vi "Detect Connected Chassis.vi"(8 "error in":errorcluster, 11 "Refnum in":refnum<k21>) -> (0 "error out":errorcluster, 2 "Chassis Information":T1[](array[typedef]) {"Modules"."Module Code" format="%.0x"})   [LabVIEW 2015, in "SMI.lvlib" / "Controller.lvclass"]
uses:
  Controller.lvclass
  Chassis/Controls/ChassisInformation.ctl
  Module/Controls/ModuleInformation.ctl
  <vilib>/nisyscfg/Close (Resources).vi
  <vilib>/nisyscfg/Close (Filter).vi
  <vilib>/nisyscfg/Close (System).vi
  <vilib>/nisyscfg/nisyscfg.lvlib
  <resource>/objmgr/niflexriosae.rc
  <resource>/objmgr/nisysapi.rc
  Module/Module.lvclass
  Chassis/Chassis.lvclass
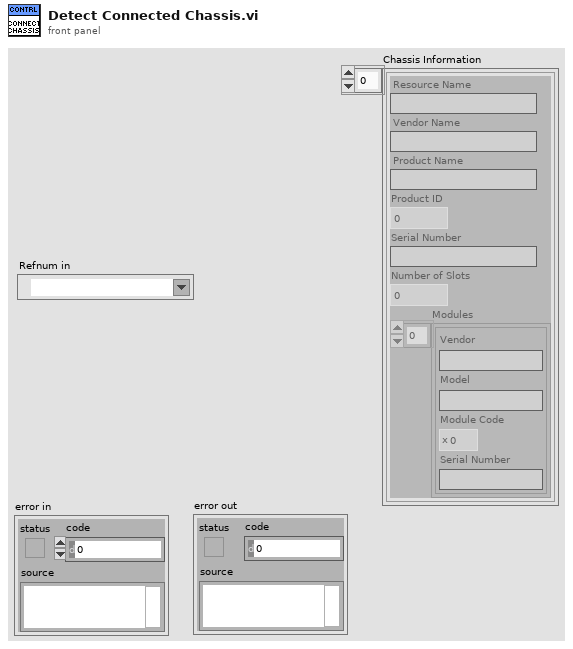
[diagram p1: front panel]
types:
  T1 = typedef "SMI.lvlib/Chassis.lvclass/ChassisInformation.ctl" = cluster{"Resource Name":string, "Vendor Name":string, "Product Name":string, "Product ID":u32, "Serial Number":string, "Number of Slots":i32, "Modules":T2[]}
  T2 = typedef "SMI.lvlib/Module.lvclass/ModuleInformation.ctl" = cluster{"Vendor":string, "Model":string, "Module Code":u32, "Serial Number":string}
  T3 = cluster{"VendorName":string, "ProdName":string, "SerialNum":string, "NumSlots":i32, "ProdID":u32, "Resource Name":string}
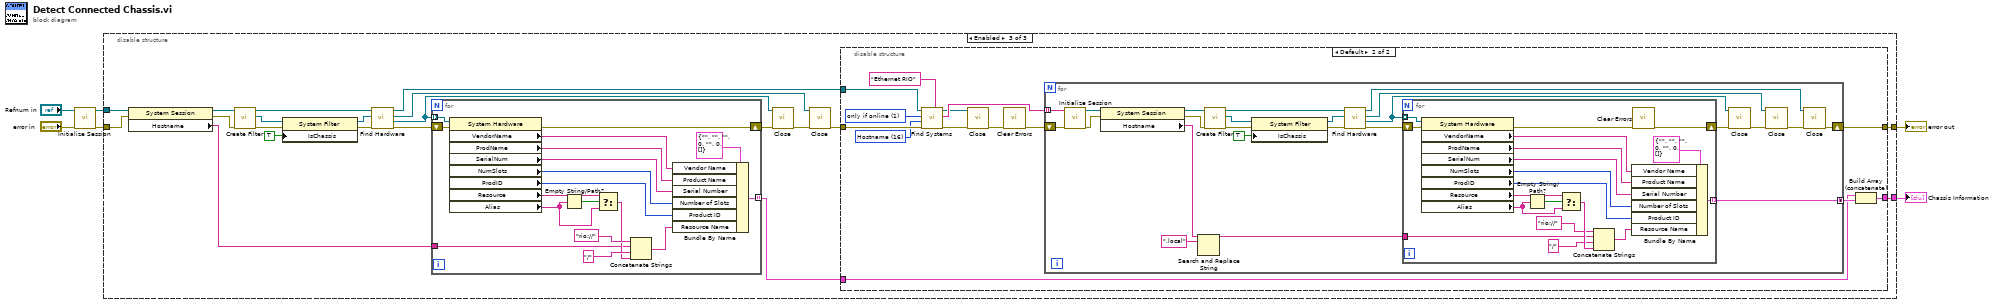
[diagram p0: block diagram]
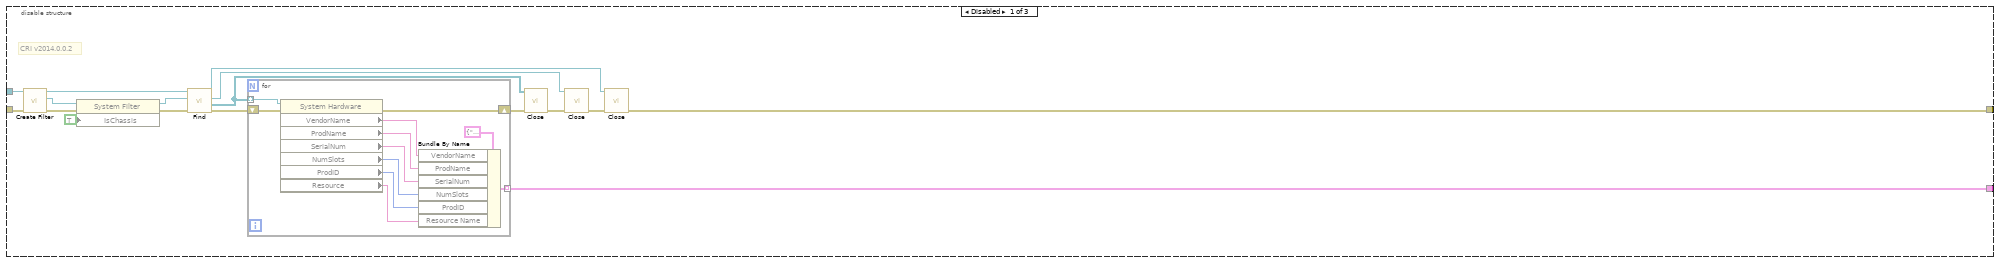
[diagram p2: hidden frame]
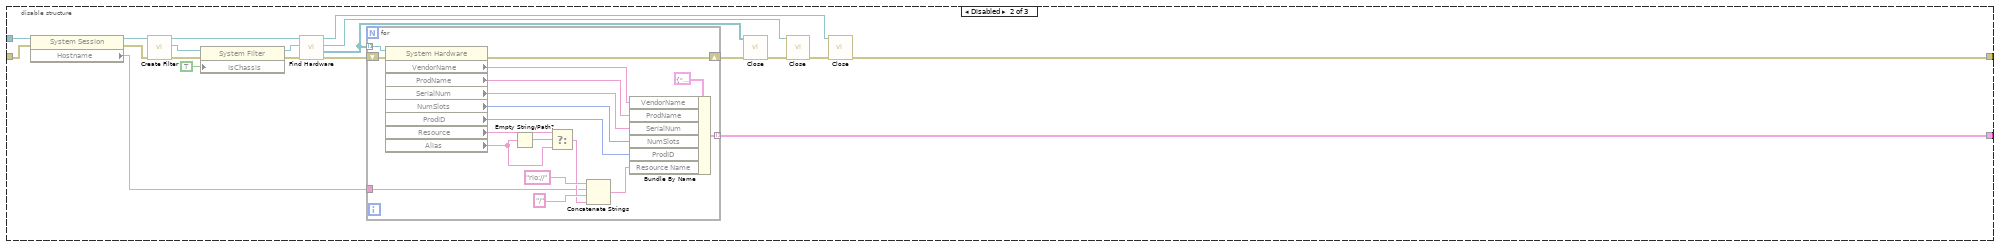
[diagram p3: hidden frame]
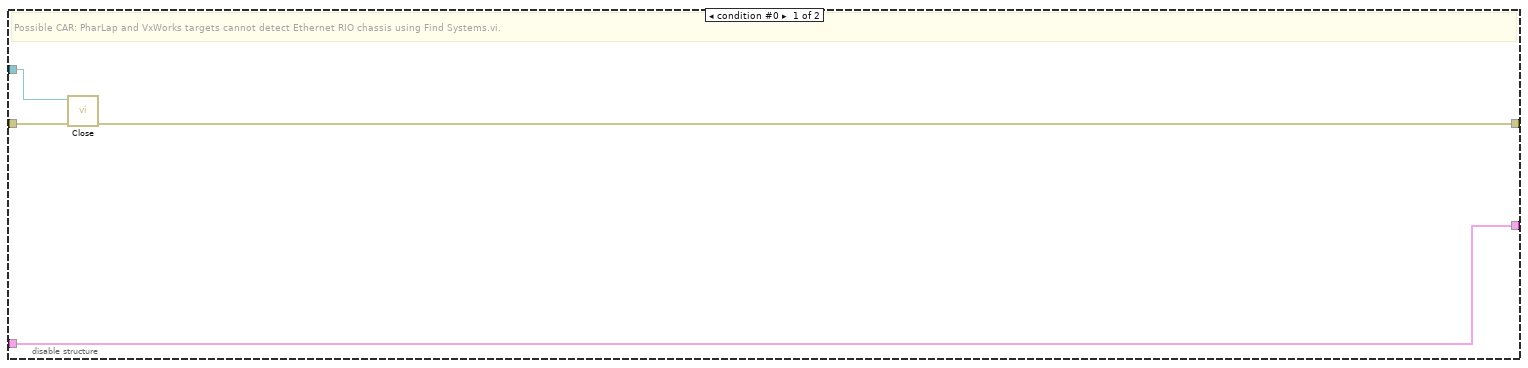
[diagram p4: hidden frame]
diagram:
  n1 = call <vilib>:"Initialize Session.vi"("error in (no error)"="error in", "Target (localhost)"="Refnum in") -> ("error out"=w3:errorcluster, "Session out"=w1:refnum<k21>)  [unwired: 8 in]
  n2 = disable-structure shown="Enabled" {
    disable-tunnel: [w17 w38 w85] -> w6
    disable-tunnel: [w16 w36 w81] -> w5
    disable-tunnel: w3 -> [w15 w40 w78]
    disable-tunnel: w1 -> [w14 w39 w80]
    frame Disabled {
      # "CRI v2014.0.0.2"
      n3 = call <vilib>:"Create Filter.vi"("error in (no error)"=w15, "Session in"=w14) -> ("error out"=w23:errorcluster, "Filter out"=w22:refnum<k20>, "Session out"=w21:refnum<k21>)  [unwired: 7 in]
      n4 = property class="System Filter"(reference=w22, error in=w23, "IsChassis"=TRUE ("Is Chassis")) -> (reference out=w20:refnum<k20>, error out=w19:errorcluster)
      n5 = call-poly <vilib>:"Find.vi"("error in (no error)"=w19, "Filter in"=w20, "Session in"=w21) -> ("error out"=w13:errorcluster, "Resources out"=w9:refnum<k20>[], "Filter out"=w8:refnum<k20>, "Session out"=w7:refnum<k21>)  [unwired: 5 in]
      n6 = for {
        tunnel: w9 -> [w34] mode=indexing
        shift-right: [w31] -> w10
        shift-left: w13 -> [w33]
        tunnel: [w32] -> w17 mode=indexing
        n7 = property class="System Hardware"(reference=w34, error in=w33) -> (error out=w31:errorcluster, "VendorName"=w29:string, "ProdName"=w28:string, "SerialNum"=w27:string, "NumSlots"=w26:i32, "ProdID"=w25:u32, "Resource"=w24:string)  [unwired: 1 out]
        n8 = Bundle By Name(cluster=T3 {"VendorName"="", "ProdName"="", "SerialNum"="", "NumSlots"=0, "ProdID"=0, "Resource Name"=""} ("cRIO_SysConfig.lvlib:Chassis Info"), "VendorName"=w29, "ProdName"=w28, "SerialNum"=w27, "NumSlots"=w26, "ProdID"=w25, "Resource Name"=w24) -> (w32:T3)
      }
      n9 = call-poly <vilib>:"Close.vi"("error in (no error)"=w10, "Resources in"=w9) -> ("error out"=w12:errorcluster)  [unwired: 9 in]
      n10 = call-poly <vilib>:"Close.vi"("error in (no error)"=w12, "Filter in"=w8) -> ("error out"=w11:errorcluster)  [unwired: 9 in]
      n11 = call-poly <vilib>:"Close.vi"("error in (no error)"=w11, "Session in"=w7) -> ("error out"=w16:errorcluster)  [unwired: 9 in]
    }
    frame Disabled {
      n12 = property class="System Session"(reference=w39, error in=w40) -> (reference out=w46:refnum<k21>, error out=w45:errorcluster, "Hostname"=w44:string)
      n13 = call <vilib>:"Create Filter.vi"("error in (no error)"=w45, "Session in"=w46) -> ("error out"=w43:errorcluster, "Filter out"=w42:refnum<k20>, "Session out"=w54:refnum<k21>)  [unwired: 7 in]
      n14 = property class="System Filter"(reference=w42, error in=w43, "IsChassis"=TRUE ("Is Chassis")) -> (reference out=w53:refnum<k20>, error out=w52:errorcluster)
      n15 = call <vilib>:"Find Hardware.vi"("error in (no error)"=w52, "Filter in"=w53, "Session in"=w54) -> ("error out"=w51:errorcluster, "Resources out"=w48:refnum<k20>[], "Filter out"=w47:refnum<k20>, "Session out"=w35:refnum<k21>)  [unwired: 5 in]
      n16 = for {
        tunnel: w48 -> [w72] mode=indexing
        shift-right: [w69] -> w49
        shift-left: w51 -> [w71]
        tunnel: [w70] -> w38 mode=indexing
        tunnel: w44 -> [w55]
        n17 = property class="System Hardware"(reference=w72, error in=w71) -> (error out=w69:errorcluster, "VendorName"=w67:string, "ProdName"=w66:string, "SerialNum"=w65:string, "NumSlots"=w64:i32, "ProdID"=w63:u32, "Resource"=w57:string, "Alias"=w58:string)  [unwired: 1 out]
        n18 = Empty String/Path?(string/path=w58) -> (empty?=w59:bool)
        n19 = Select(t=w57, s=w59, f=w58) -> (s? t:f=w56:string)
        n20 = Concatenate Strings("rio://" ("string"), w55, "/" ("string"), w56) -> (w62:string)
        n21 = Bundle By Name(cluster=T3 {"VendorName"="", "ProdName"="", "SerialNum"="", "NumSlots"=0, "ProdID"=0, "Resource Name"=""} ("cRIO_SysConfig.lvlib:Chassis Info"), "VendorName"=w67, "ProdName"=w66, "SerialNum"=w65, "NumSlots"=w64, "ProdID"=w63, "Resource Name"=w62) -> (w70:T3)
      }
      n22 = call-poly <vilib>:"Close.vi"("error in (no error)"=w49, "Resources in"=w48) -> ("error out"=w50:errorcluster)  [unwired: 9 in]
      n23 = call-poly <vilib>:"Close.vi"("error in (no error)"=w50, "Filter in"=w47) -> ("error out"=w37:errorcluster)  [unwired: 9 in]
      n24 = call-poly <vilib>:"Close.vi"("error in (no error)"=w37, "Session in"=w35) -> ("error out"=w36:errorcluster)  [unwired: 9 in]
    }
    frame Enabled {
      n25 = property class="System Session"(reference=w80, error in=w78) -> (reference out=w79:refnum<k21>, error out=w77:errorcluster, "Hostname"=w76:string)
      n26 = call <vilib>:"Create Filter.vi"("error in (no error)"=w77, "Session in"=w79) -> ("error out"=w75:errorcluster, "Filter out"=w74:refnum<k20>, "Session out"=w93:refnum<k21>)  [unwired: 7 in]
      n27 = property class="System Filter"(reference=w74, error in=w75, "IsChassis"=TRUE ("Is Chassis")) -> (reference out=w92:refnum<k20>, error out=w91:errorcluster)
      n28 = call <vilib>:"Find Hardware.vi"("error in (no error)"=w91, "Filter in"=w92, "Session in"=w93) -> ("error out"=w90:errorcluster, "Resources out"=w87:refnum<k20>[], "Filter out"=w86:refnum<k20>, "Session out"=w82:refnum<k21>)  [unwired: 5 in]
      n29 = for {
        tunnel: w87 -> [w172] mode=indexing
        shift-right: [w169] -> w88
        shift-left: w90 -> [w171]
        tunnel: [w170] -> w84 mode=indexing
        tunnel: w76 -> [w156]
        n30 = property class="System Hardware"(reference=w172, error in=w171) -> (error out=w169:errorcluster, "VendorName"=w168:string, "ProdName"=w167:string, "SerialNum"=w166:string, "NumSlots"=w165:i32, "ProdID"=w164:u32, "Resource"=w158:string, "Alias"=w159:string)  [unwired: 1 out]
        n31 = Empty String/Path?(string/path=w159) -> (empty?=w160:bool)
        n32 = Select(t=w158, s=w160, f=w159) -> (s? t:f=w157:string)
        n33 = Concatenate Strings("rio://" ("string"), w156, "/" ("string"), w157) -> (w163:string)
        n34 = Bundle By Name(cluster=T1 {"Resource Name"="", "Vendor Name"="", "Product Name"="", "Product ID"=0, "Serial Number"="", "Number of Slots"=0, "Modules"=[]} ("Chassis Information"), "Vendor Name"=w168, "Product Name"=w167, "Serial Number"=w166, "Number of Slots"=w165, "Product ID"=w164, "Resource Name"=w163) -> (w170:T1)
      }
      n35 = call-poly <vilib>:"Close.vi"("error in (no error)"=w88, "Resources in"=w87) -> ("error out"=w89:errorcluster)  [unwired: 9 in]
      n36 = call-poly <vilib>:"Close.vi"("error in (no error)"=w89, "Filter in"=w86) -> ("error out"=w83:errorcluster)  [unwired: 9 in]
      n37 = disable-structure shown="Default" {
        disable-tunnel: [w94 w110] -> w85
        disable-tunnel: w84 -> [w94 w109]
        disable-tunnel: w83 -> [w97 w108]
        disable-tunnel: w82 -> [w96 w107]
        disable-tunnel: [w95 w105] -> w81
        frame condition #0 {
          # "Possible CAR: PharLap and VxWorks targets cannot detect Ethernet RIO chassis using Find Systems.vi."
          n38 = call-poly <vilib>:"Close.vi"("error in (no error)"=w97, "Session in"=w96) -> ("error out"=w95:errorcluster)  [unwired: 9 in]
        }
        frame condition #1 (active) {
          w101 = u32 1 items=["none"=0, "only if online"=1, "all"=3] ("Include Cached Results (all)")
          w102 = u32 16 items=["Hostname"=16, "Hostname (IP)"=18, "Hostname (MAC)"=19, "IP"=32, "IP (Hostname)"=33, "IP (MAC)"=35, "MAC"=48, "MAC (Hostname)"=49, "MAC (IP)"=50] ("Output (Hostname and IP)")
          n39 = call <vilib>:"Find Systems.vi"("Device Class"="Ethernet RIO", "error in (no error)"=w108, "Output (Hostname and IP)"=w102, "Include Cached Results (all)"=w101, "Session in (localhost)"=w107) -> ("error out"=w104:errorcluster, "Detected Systems"=w106:string[], "Session out"=w103:refnum<k21>)  [unwired: 4 in]
          n40 = call-poly <vilib>:"Close.vi"("error in (no error)"=w104, "Session in"=w103) -> ("error out"=w99:errorcluster)  [unwired: 9 in]
          n41 = call <vilib>:"Clear Errors.vi"("error in (no error)"=w99) -> ("error out"=w98:errorcluster)  [unwired: 5 in, 1 out]
          n42 = for {
            shift-right: [w124] -> w105
            shift-left: w98 -> [w135]
            tunnel: [w126] -> w111 mode=concatenating
            tunnel: w106 -> [w122] mode=indexing
            n43 = call <vilib>:"Initialize Session.vi"("error in (no error)"=w135, "Target (localhost)"=w122) -> ("error out"=w119:errorcluster, "Session out"=w121:refnum<k21>)  [unwired: 8 in]
            n44 = property class="System Session"(reference=w121, error in=w119) -> (reference out=w120:refnum<k21>, error out=w118:errorcluster, "Hostname"=w117:string)
            n45 = Search and Replace String(input string=w117, search string=".local") -> (result string=w116:string)  [unwired: 6 in, 3 out]
            n46 = call <vilib>:"Create Filter.vi"("error in (no error)"=w118, "Session in"=w120) -> ("error out"=w112:errorcluster, "Filter out"=w113:refnum<k20>, "Session out"=w127:refnum<k21>)  [unwired: 7 in]
            n47 = property class="System Filter"(reference=w113, error in=w112, "IsChassis"=TRUE ("Is Chassis")) -> (reference out=w128:refnum<k20>, error out=w129:errorcluster)
            n48 = call <vilib>:"Find Hardware.vi"("error in (no error)"=w129, "Filter in"=w128, "Session in"=w127) -> ("error out"=w130:errorcluster, "Resources out"=w133:refnum<k20>[], "Filter out"=w134:refnum<k20>, "Session out"=w125:refnum<k21>)  [unwired: 5 in]
            n49 = for {
              tunnel: w133 -> [w154] mode=indexing
              shift-right: [w145] -> w132
              shift-left: w130 -> [w153]
              tunnel: [w152] -> w126 mode=indexing
              tunnel: w116 -> [w137]
              n50 = property class="System Hardware"(reference=w154, error in=w153) -> (error out=w146:errorcluster, "VendorName"=w151:string, "ProdName"=w150:string, "SerialNum"=w149:string, "NumSlots"=w148:i32, "ProdID"=w147:u32, "Resource"=w139:string, "Alias"=w138:string)  [unwired: 1 out]
              n51 = Empty String/Path?(string/path=w138) -> (empty?=w143:bool)
              n52 = Select(t=w139, s=w143, f=w138) -> (s? t:f=w144:string)
              n53 = Concatenate Strings("rio://" ("string"), w137, "/" ("string"), w144) -> (w140:string)
              n54 = Bundle By Name(cluster=T1 {"Resource Name"="", "Vendor Name"="", "Product Name"="", "Product ID"=0, "Serial Number"="", "Number of Slots"=0, "Modules"=[]} ("Chassis Information"), "Vendor Name"=w151, "Product Name"=w150, "Serial Number"=w149, "Number of Slots"=w148, "Product ID"=w147, "Resource Name"=w140) -> (w152:T1)
              n55 = call <vilib>:"Clear Errors.vi"("error in (no error)"=w146) -> ("error out"=w145:errorcluster)  [unwired: 5 in, 1 out]
            }
            n56 = call-poly <vilib>:"Close.vi"("error in (no error)"=w132, "Resources in"=w133) -> ("error out"=w131:errorcluster)  [unwired: 9 in]
            n57 = call-poly <vilib>:"Close.vi"("error in (no error)"=w131, "Filter in"=w134) -> ("error out"=w123:errorcluster)  [unwired: 9 in]
            n58 = call-poly <vilib>:"Close.vi"("error in (no error)"=w123, "Session in"=w125) -> ("error out"=w124:errorcluster)  [unwired: 9 in]
          }
          n59 = Build Array (concatenate)(w109, w111) -> (w110:T1[])
        }
      }
    }
  }
  "error out" <- w5
  "Chassis Information" <- w6
